vi "3.0-Global.vi"() -> ()   [LabVIEW 2010]
doc: "This global exits on the RT target and is for passing data between the parallel loops. This could also be achieved by queues, but for most data a queue is more work than it is worth-massive overkill to tell the act loop to turn left. If you want to tell the act loop the distance it can go in any of 4000 different paths and the error bars on each number then you do not want to use the global variables. instead you should reconsider your algorithm or, if the massive data is really neccissary come up with a way to share the memory. Find out how laview deals with pointers, deal with the data through a shared subvi et cetera..."
uses:
  4-High Neurons/4.6.1-Action Neuron Typedef.ctl
  6-OCU Neurons/6.1-UDP Saitek.ctl
  4-High Neurons/Current GPS Data.ctl
  3.1-Where/3.1.1-VectorNav/3.1.1-VectorNav Data.ctl
  3.1-Where/3.1.1-VectorNav/3.1.1-VectorNav Command Type.ctl
panel:
  out "Stop Loops":bool
  in  "Tabs, For Convenience":T1(tab)
  in  "GPS VISA resource name":refnum<visa-resource-name>="ASRL1::INSTR"
  in  "4.1.1-VectorNav Data":T2
  out "GPS Data":T3 {"Longitude (dd.mmmmmm)" format="%#.6g"; "Lattitude (dd.mmmmmm)" format="%#.6g"}
  in  "4.1.1-VectorNav Cmd":T4
  in  "4.2 18 Paths":dbl[](array[numeric])
  in  "4.1.1-VectorNav Status":string
  out "Joystick Data":T5 {"Right" scale=-32767.0..32767.0; "Left" scale=-32767.0..32767.0; "Yaw" scale=-32767.0..32767.0; "Roll" scale=-32767.0..32767.0; "Pitch" scale=-32767.0..32767.0}
  in  "4.6 Joystick Act Neurons":T6
  out "4.6 Lidar Declination, Deg":dbl
  out "4.6 Drive Speed, Mph":dbl
  out "4.6 Steering Angle, Deg":dbl
  out "4.6 HB":bool
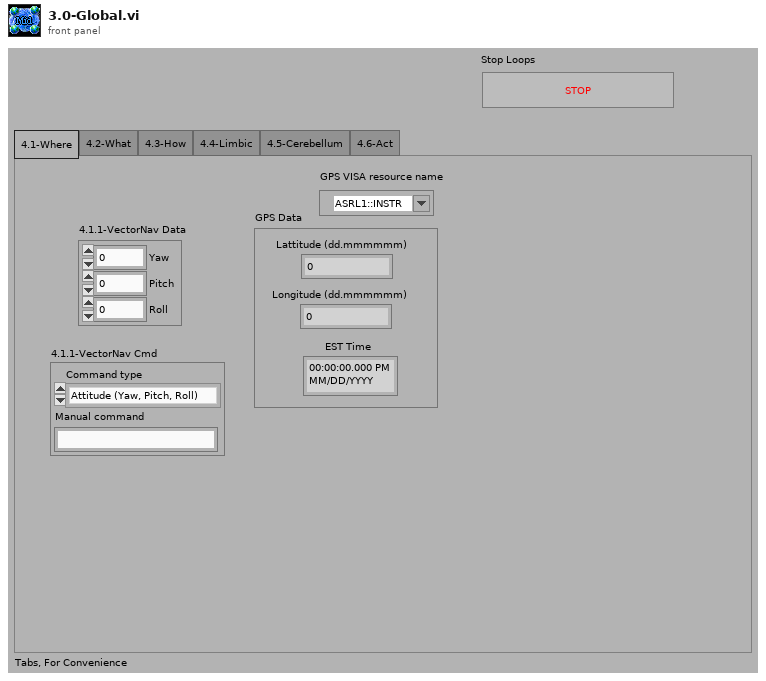
[diagram p1: front panel]
types:
  T1 = enum32{"4.1-Where", "4.2-What", "4.3-How", "4.4-Limbic", "4.5-Cerebellum", "4.6-Act"}
  T2 = typedef "3.1.1-VectorNav Data.ctl" = cluster{"Yaw":dbl, "Pitch":dbl, "Roll":dbl}
  T3 = typedef "Current GPS Data.ctl" = cluster{"Lattitude (dd.mmmmmm)":dbl, "Longitude (dd.mmmmmm)":dbl, "EST Time":timestamp}
  T4 = typedef "3.1.1-VectorNav Command Type.ctl" = cluster{"Command type":enum16{"Attitude (Yaw, Pitch, Roll)", "Write Current Settings", "Disable Async Output", "Tare", "Manual"}, "Manual command":string}
  T5 = typedef "6.1-UDP Saitek.ctl" = cluster{"Trig":bool, "2":bool, "3":bool, "4":bool, "5":bool, "6":bool, "7":bool, "8":bool, "9":bool, "10":bool, "11":bool, "Pitch":i32, "Ang":bool[], "Wheel":dbl, "Roll":i32, "Yaw":i32, "Left":i32, "Right":i32}
  T6 = typedef "4.6.1-Action Neuron Typedef.ctl" = cluster{"AutoSubsume?":bool, "Fuzzy Legitimacy":dbl, "Directional Functionality":dbl[], "Inhibit All Motors?":bool, "Directional Legitimacy":u8[]}
diagram:
